vi "ReadCtrlAttrListGen.vi"(4 "Error in":errorcluster, 7 "Attribut":string="DisAtStartup") -> (0 "Error out":errorcluster, 1 "SousTitres":string[](array[string]), 2 "Étiquette":string[](array[string]), 3 "Controls Out":refnum<vi>[](array[refnum]))   [LabVIEW 2010]
doc: "Ce VI ouvre le fichier de sauvegarde des modèles et lit les positions du modèle spécifié."
uses:
  <vilib>/Utility/config.llb/Read Key (String).vi
  <vilib>/Utility/config.llb/NI_LVConfig.lvlib
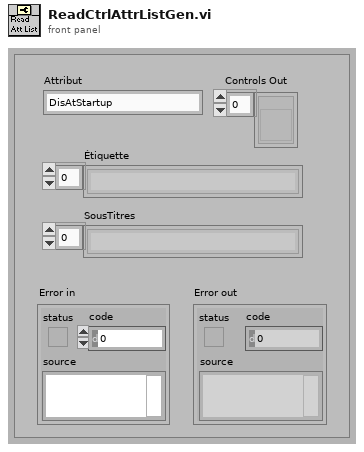
[diagram p1: front panel]
types:
  T1 = typedef "NI_LVConfig.lvlib/Config Data RefNum.ctl" = refnum<k1>
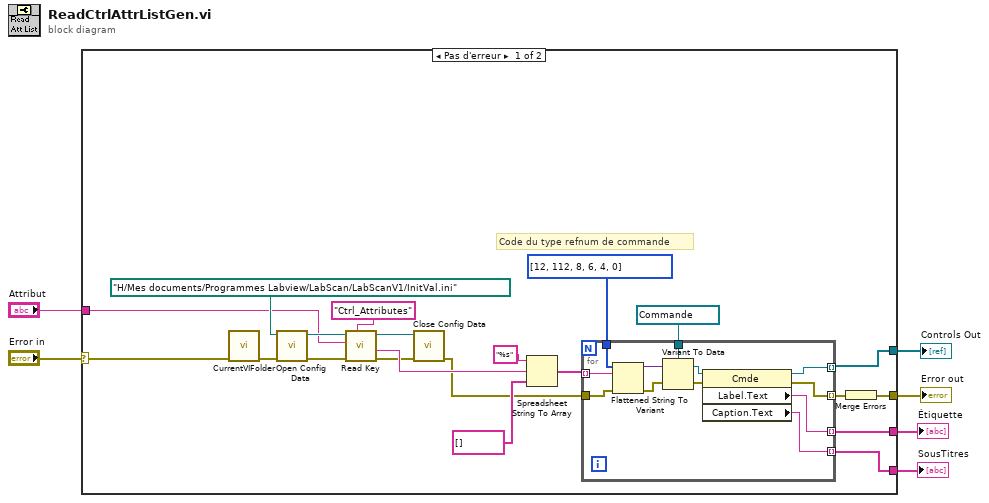
[diagram p0: block diagram]
diagram:
  n1 = case shown="Pas d'erreur" "Error in" {
    selector: "Error in" -> [w13 w40]
    tunnel: [w7 w40] -> w6
    tunnel: [w16 _] -> w4
    tunnel: [w15 _] -> w3
    tunnel: [w14 _] -> w2
    tunnel: "Attribut" -> [w10 _]
    frame No Error {
      # "Code du type refnum de commande"
      n2 = call <userlib>:"CurrentVIFolder.vi"("error in (no error)"=w13) -> ("error out"=w27:errorcluster)  [unwired: 8 in, 2 out]
      n3 = call <vilib>:"Open Config Data.vi"("error in (no error)"=w27, "configuration file path"=path "H:/Mes documents/Programmes Labview/LabScan/LabScanV1/InitVal.ini" ("chemin du VI")) -> ("error out"=w12:errorcluster, "refnum"=w25:T1)  [unwired: 7 in, 1 out]
      n4 = call-poly <vilib>:"Read Key.vi"("section"="Ctrl_Attributes", "error in (no error)"=w12, "key"=w10, "refnum"=w25) -> ("error out"=w11:errorcluster, "value"=w21:string, "refnum out"=w23:T1)  [unwired: 4 in, 1 out]
      n5 = call <vilib>:"Close Config Data.vi"("error in (no error)"=w11, "refnum"=w23) -> ("error out"=w9:errorcluster)  [unwired: 8 in, 1 out]
      n6 = Spreadsheet String To Array(format string="%s" ("chaîne de format"), spreadsheet string=w21, array type (2D Dbl)=string[] []) -> (array=w19:string[])  [unwired: 1 in]
      n7 = for {
        tunnel: w19 -> [w39] mode=indexing
        tunnel: refnum<vi> refnum ("référence") -> [w36]
        tunnel: [w28] -> w16 mode=indexing
        tunnel: [w34] -> w15 mode=indexing
        tunnel: i16[] [12, 112, 8, 6, 4, 0] ("chaîne de type 2") -> [w33]
        tunnel: [w32] -> w14 mode=indexing
        tunnel: w9 -> [w31]
        tunnel: [w29] -> w8 mode=indexing
        n8 = Flattened String To Variant(4:w31, 6:w39, 7:w33) -> (0:w37:errorcluster, 3:w38:variant)
        n9 = Variant To Data(error in=w37, Variant=w38, type=w36) -> (error out=w30:errorcluster, data=w35:refnum<vi>)
        n10 = property class="Cmde"(reference=w35, error in=w30) -> (reference out=w28:refnum<vi>, error out=w29:errorcluster, "Label.Text"=w34:string, "Caption.Text"=w32:string)
      }
      n11 = Merge Errors(w8) -> (w7:errorcluster)
    }
    frame Error {
    }
  }
  "Error out" <- w6
  "Controls Out" <- w4
  "Étiquette" <- w3
  "SousTitres" <- w2
